vi "http_post_get.vi"(6 "LabVIEW Web Service":refnum<class "Web Service.lvclass">) -> ()   [LabVIEW 2021]
uses:
  <vilib>/wsapi/Web Service.lvclass
  <vilib>/httpClient/LabVIEWHTTPClient.lvlib
  <vilib>/httpClient/POSTBuffer.vi
panel:
  out "body 2":string
  out "headers 2":string
  out "body":string
  out "headers":string
  # "Use the web service input terminal to call the VIs on the Service subpalette of the Web Services palette. Do not remove it from the connector pane unless you don't need access to the palette."
  # "Any additional terminals added to the connector pane of a startup VI will be ignored."
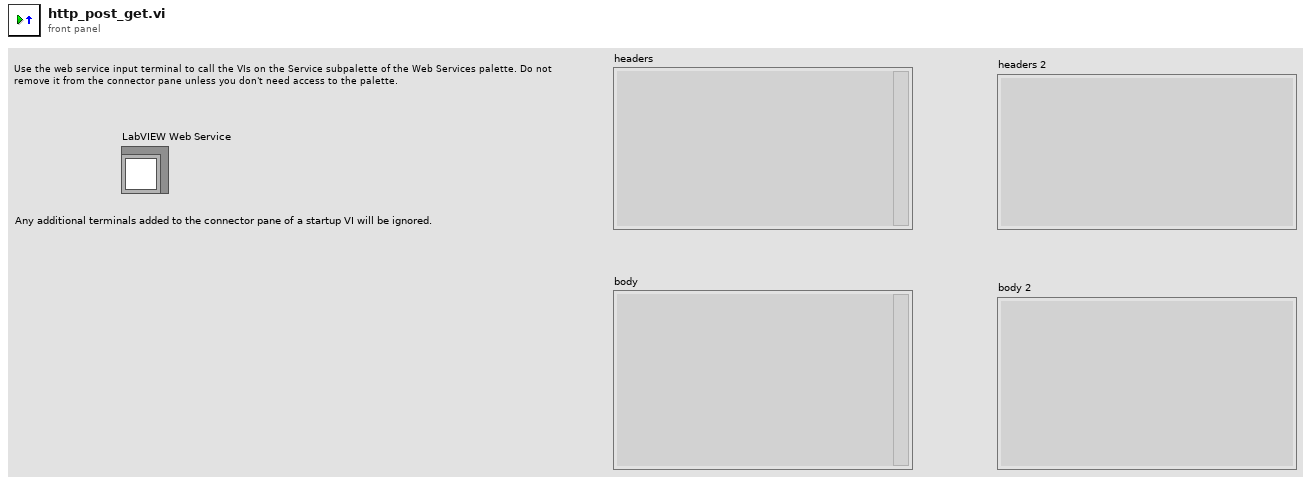
[diagram p1: front panel]
types:
  T1 = typedef "LabVIEWHTTPClient.lvlib/ClientHandle.ctl" = refnum<k1>
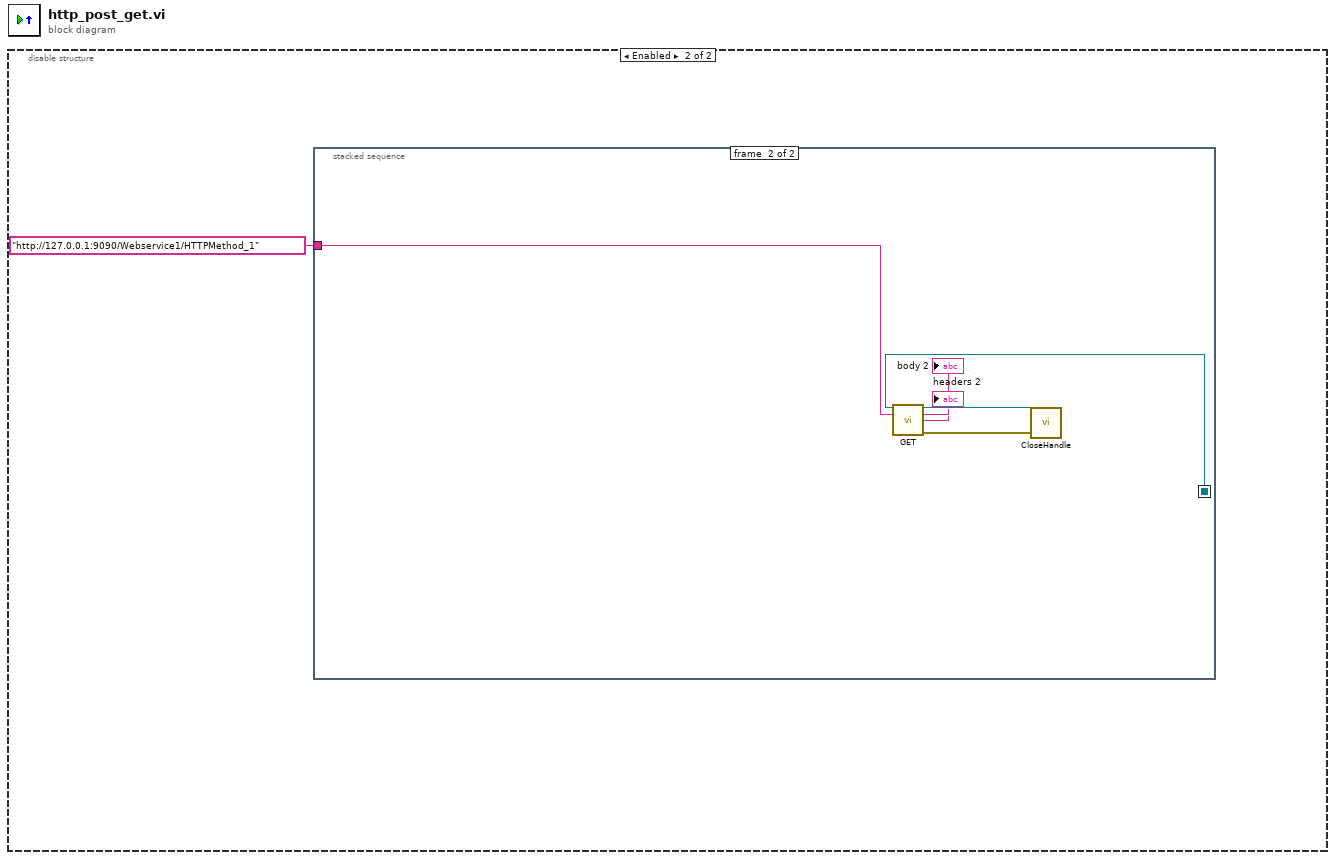
[diagram p0: block diagram]
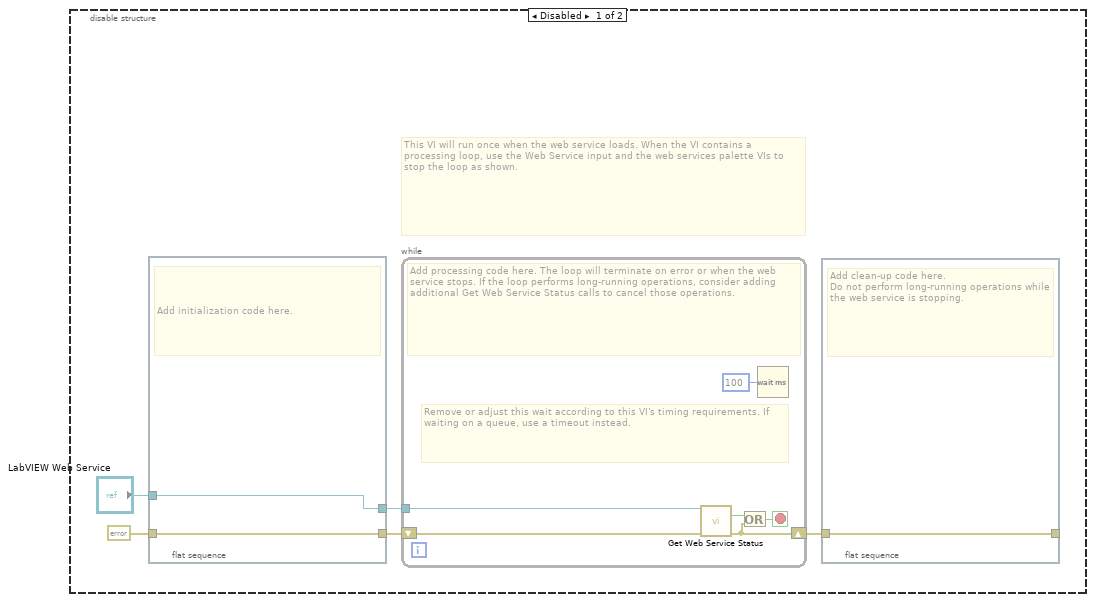
[diagram p2: hidden frame]
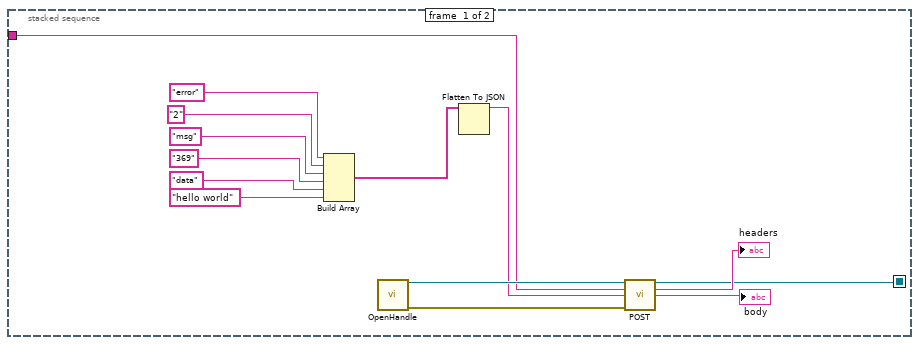
[diagram p3: hidden frame]
diagram:
  n1 = disable-structure shown="Enabled" {
    frame Disabled {
      # "This VI will run once when the web service loads. When the VI contains a processing loop, use the Web Service input and the web services palette VIs to stop the loop as shown."
      n2 = flat-sequence {
        tunnel: "LabVIEW Web Service" -> [w8]
        tunnel: [w8] -> w4
        tunnel: [w7] -> w3
        tunnel: errorcluster {"status"=FALSE, "code"=0, "source"=""} ("error constant") -> [w7]
        frame #0 {
          # "Add initialization code here."
        }
      }
      n3 = while {
        tunnel: w4 -> [w13]
        shift-right: [w10] -> w1
        shift-left: w3 -> [w11]
        stop <- w12 stop-if-true
        # "Remove or adjust this wait according to this VI's timing requirements. If waiting on a queue, use a timeout instead."
        # "Add processing code here. The loop will terminate on error or when the web service stops. If the loop performs long-running operations, consider adding additional Get Web Service Status calls to cancel those operations."
        n4 = call <vilib>:"Get Web Service Status.vi"("LabVIEW Web Service"=w13, "error in (no error)"=w11) -> ("service stopping?"=w14:bool, "error out"=w10:errorcluster)  [unwired: 11 in, 1 out]
        n5 = Or(x=w14, y=w10) -> (x .or. y?=w12:bool)
        n6 = Wait (ms)(milliseconds to wait=u32 100) -> ()  [unwired: 1 out]
      }
      n7 = flat-sequence {
        tunnel: [w6] -> _
        tunnel: w1 -> [w6]
        frame #0 {
          # "Add clean-up code here.\nDo not perform long-running operations while the web service is stopping."
        }
      }
    }
    frame Enabled {
      n8 = stacked-sequence {
        seq-local: [w17 _] -> [_ w34]
        tunnel: "http://127.0.0.1:9090/Webservice1/HTTPMethod_1" -> [w16 w35]
        frame #0 {
          n9 = Build Array("error", "2", "msg", "369", "data", "hello world") -> (w23:string[])
          n10 = call <vilib>:"OpenHandle.vi"() -> ("client handle out"=w22:T1, "error out"=w21:errorcluster)  [unwired: 14 in]
          n11 = Flatten To JSON(anything=w23) -> (JSON string=w20:string)  [unwired: 2 in, 1 out]
          n12 = call-poly <vilib>:"POST.vi"("client handle"=w22, "url"=w16, "buffer"=w20, "error in (no error)"=w21) -> ("client handle out"=w17:T1, "headers"=→"headers":string, "body"=→"body":string)  [unwired: 8 in, 1 out]
        }
        frame #1 {
          n13 = call <vilib>:"GET.vi"("client handle"=w34, "url"=w35) -> ("client handle out"=w33:T1, "headers"=→"headers 2":string, "body"=→"body 2":string, "error out"=w32:errorcluster)  [unwired: 10 in]
          n14 = call <vilib>:"CloseHandle.vi"("client handle"=w33, "error in (no error)"=w32) -> ()  [unwired: 13 in, 1 out]
        }
      }
    }
  }
